vi "test-diff-drive-voltage-constraint.vi"(8 "error in (no error)":errorcluster) -> (0 "error out 4":errorcluster, 3 "Test Passed":bool)   [LabVIEW 2019]
uses:
  <vilib>/Rock Robotics/WPI/ThirdParty/JAS_Junk/TrajLib/POSE2D.ctl
  <vilib>/Rock Robotics/WPI/ThirdParty/JAS_Junk/TrajLib/TRANSLATION2D.ctl
  <vilib>/Rock Robotics/WPI/ThirdParty/JAS_Junk/TrajLib/ROTATION2D.ctl
  <vilib>/Rock Robotics/WPI/ThirdParty/JAS_Junk/TrajLib/TRAJECTORY_SPLINE_TYPE_ENUM.ctl
  <vilib>/Rock Robotics/WPI/ThirdParty/JAS_Junk/TrajLib/Translation_Create.vi
  <vilib>/Rock Robotics/WPI/ThirdParty/JAS_Junk/TrajLib/Rotation_CreateAngle.vi
  <vilib>/Rock Robotics/SystemInterfaces/NetworkCommunication/NetComm_UsageReport_report.vi
  <vilib>/Rock Robotics/WPI/ThirdParty/JAS_Junk/TrajLib/DiffDriveVoltageConstraint_New.vi
  <vilib>/Rock Robotics/WPI/ThirdParty/JAS_Junk/TrajLib/Util_LibraryGlobals.vi
  <vilib>/Rock Robotics/WPI/ThirdParty/JAS_Junk/TrajLib/Trajectory_Library.lvlib
panel:
  out "Accl Limit":dbl
  out "Abs chassis Accel":cluster{dbl[], dbl[]}[](graph)
  out "error out 3":errorcluster
  out "error out 2":errorcluster
  in  "Max Voltage-Test2":dbl=10.0 format="%#_13g"
  out "Motor VOltage Vs Time":cluster{dbl[], dbl[]}[](graph)
  in  "Max Voltage":dbl=10.0 format="%#_13g"
  out "Min Right":dbl
  out "min Left":dbl
  out "Left <":bool
  out "Left >":bool
  out "Right <":bool
  out "Right >":bool
  out "Max Right":dbl
  out "max Left":dbl
  out "Position Graph":cluster{dbl[], dbl[]}[](graph)
  out "Waypoints":T1[](array[typedef]) {"ROTATION"."SIN" format="%13.4f"; "ROTATION"."COS" format="%13.4f"; "ROTATION"."VALUE" format="%13.4f"; "TRANSLATION"."Y" format="%14.3f"; "TRANSLATION"."X" format="%14.3f"}
  out "TotalTImeSecs":dbl
  out "Error":bool
  out "error out":errorcluster
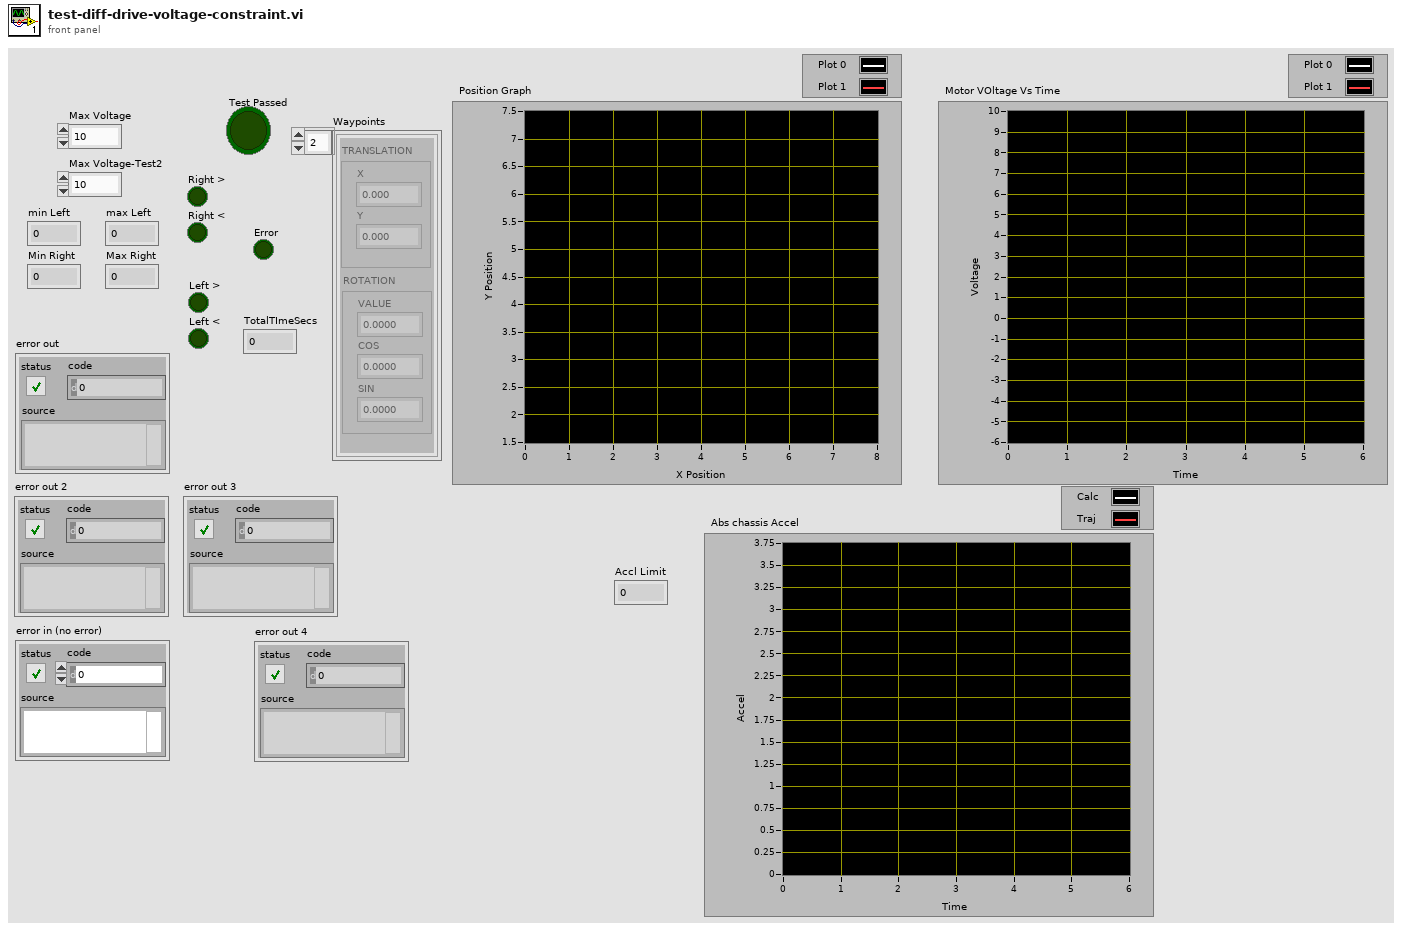
[diagram p1: front panel]
types:
  T1 = typedef "Trajectory_Library.lvlib/POSE2D.ctl" = cluster{"TRANSLATION":T2, "ROTATION":T3}
  T2 = typedef "Trajectory_Library.lvlib/TRANSLATION2D.ctl" = cluster{"X":dbl, "Y":dbl}
  T3 = typedef "Trajectory_Library.lvlib/ROTATION2D.ctl" = cluster{"VALUE":dbl, "COS":dbl, "SIN":dbl}
  T4 = typedef "Trajectory_Library.lvlib/TRAJECTORY_SPLINE_TYPE_ENUM.ctl" = enum16{"Cubic", "Cubic With Weights", "Quintic", "Quintic With Weights"}
  T5 = typedef "Trajectory_Library.lvlib/TRAJ_CONFIG.ctl" = cluster{"MaxVelocity":dbl, "Max Acceleration":dbl, "StartVelocity":dbl, "End Velocity":dbl, "Reversed":bool, "DiffDrKineConstntDefined":bool, "CentAcellConstntDefined":bool, "DiffDrVoltConstntDefined":bool, "DIFF_DRIVE_KINE_CONSTRAINT":T6, "CENTRIPETAL_ACCEL_CONSTRAINT":T8, "SwerveDrKineConstntDefined":bool, "SWERVE_DRIVE_KINE_CONSTRAINT":T9, "DIFF_DRIVE_VOLTAGE_CONSTRAINT":T12, "MECANUM_DRIVE_KINE_CONSTRAINT":T14, "MecanumDrKineConstntDefined":bool}
  T6 = typedef "Trajectory_Library.lvlib/TRAJ_CONSTRAINT_DIIF_DRIVE_KINEMATICS.ctl" = cluster{"Max Speed (M/S)":dbl, "DIFF_DRIVE_KINEMATICS":T7, "Max Accel (M/S2)":dbl}
  T7 = typedef "Trajectory_Library.lvlib/DIFF_DRIVE_KINEMATICS.ctl" = cluster{"TrackWidth_Meters":dbl}
  T8 = typedef "Trajectory_Library.lvlib/TRAJ_CONSTRAINT_CENTRIPETAL_ACCEL.ctl" = cluster{"Max Cent Accel":dbl}
  T9 = typedef "Trajectory_Library.lvlib/TRAJ_CONSTRAINT_SWERVE_DRIVE_KINEMATICS.ctl" = cluster{"Max Speed (M/S)":dbl, "SwerveKinematics":T10}
  T10 = typedef "Trajectory_Library.lvlib/SWERVE_DRIVE_KINEMATICS.ctl" = cluster{"NumModules":i32, "InverseKinematics":T11, "ForwardKinematics":T11, "Modules":T2[], "PrevCoR":T2}
  T11 = typedef "NI_Matrix.lvlib/RealMatrix.ctl" = dbl[][]
  T12 = typedef "Trajectory_Library.lvlib/TRAJ_CONSTRAINT_DIIF_DRIVE_VOLTAGE.ctl" = cluster{"Max Voltage":dbl, "DIFF_DRIVE_KINEMATICS":T7, "SIMPLE_MOTOR_FF":T13}
  T13 = typedef "Trajectory_Library.lvlib/SIMPLE_MOTOR_FF.ctl" = cluster{"Ks":dbl, "Kv":dbl, "Ka":dbl}
  T14 = typedef "Trajectory_Library.lvlib/TRAJ_CONSTRAINT_MECA_DRIVE_KINEMATICS.ctl" = cluster{"Max Speed (M/S)":dbl, "MECA_DRIVE_KINEMATICS":T15}
  T15 = typedef "Trajectory_Library.lvlib/MECA_DRIVE_KINEMATICS.ctl" = cluster{"FrontLeft":T2, "FrontRight":T2, "RearLeft":T2, "RearRight":T2, "InverseKinematics":T11, "ForwardKinematics":T11, "PrevCoR":T2}
  T16 = typedef "Trajectory_Library.lvlib/WEIGHTED_WAYPOINT.ctl" = cluster{"TRANSLATION":T2, "ROTATION":T3, "SCALAR":dbl}
  T17 = typedef "Trajectory_Library.lvlib/TRAJECTORY.ctl" = cluster{"TotalTImeSecs":dbl, "States":T18[]}
  T18 = typedef "Trajectory_Library.lvlib/TRAJ_STATE.ctl" = cluster{"TimeSeconds":dbl, "Velocity":dbl, "Acceleration":dbl, "POSE":T1, "Curvature":dbl}
  T19 = typedef "Trajectory_Library.lvlib/CHASSIS_SPEEDS.ctl" = cluster{"vX":dbl, "vY":dbl, "vOmega":dbl}
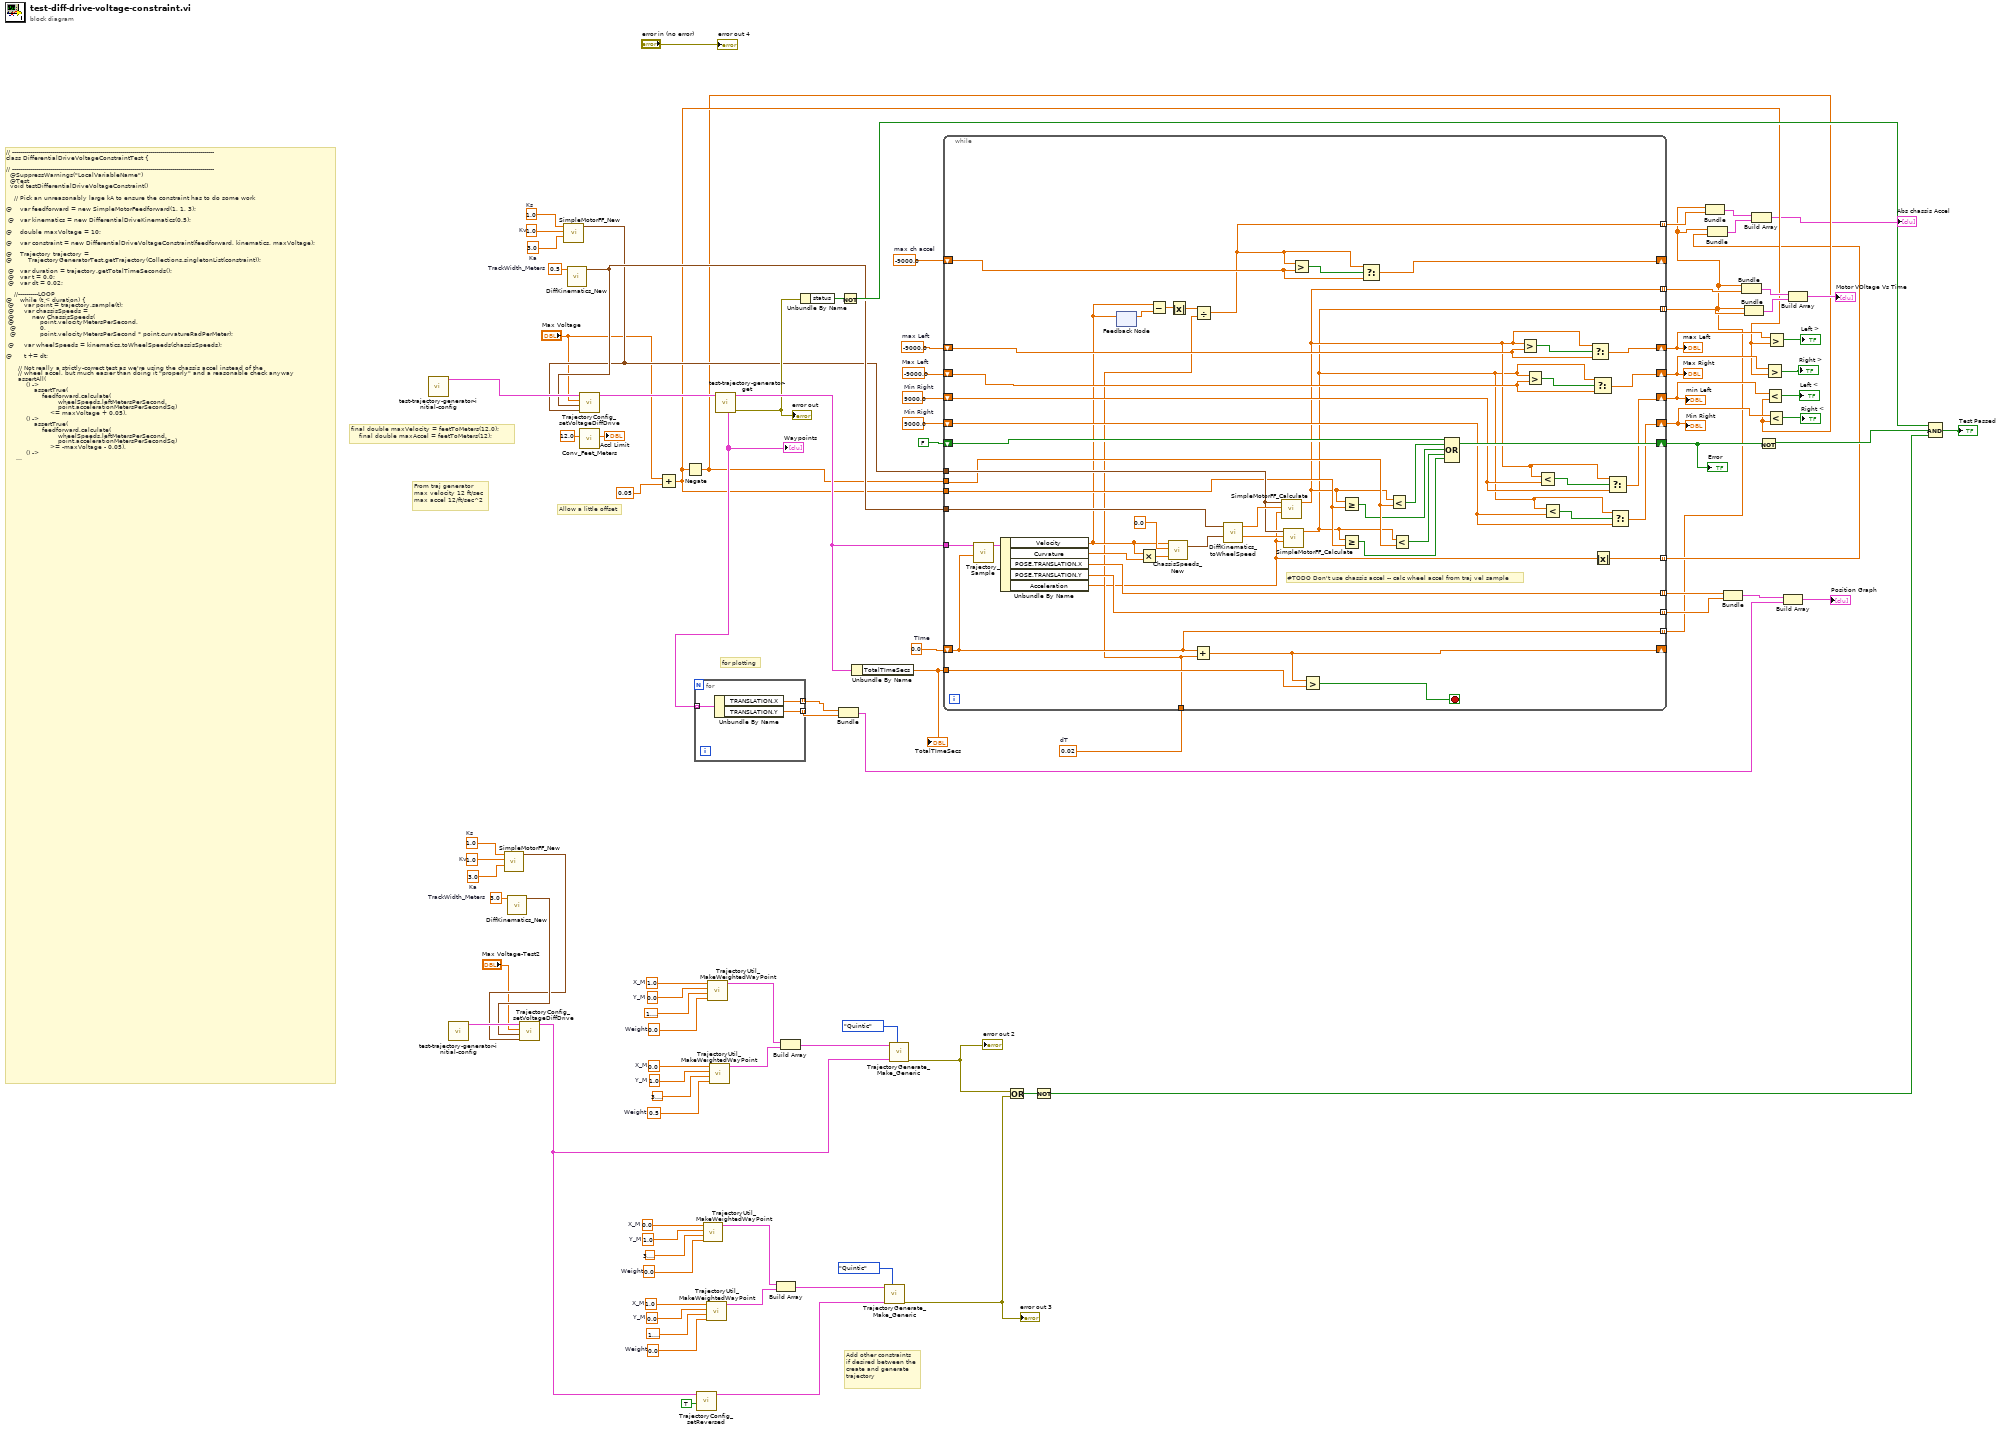
[diagram p0: block diagram]
diagram:
  w9 = -9000.0  # max ch accel
  w32 = 1.0  # X_M
  w31 = 0.0  # Y_M
  w30 = 0.0  # Weight
  w29 = 0.0  # X_M
  w28 = 1.0  # Y_M
  w27 = 0.0  # Weight
  w41 = 0.0  # X_M
  w40 = 1.0  # Y_M
  w39 = 0.5  # Weight
  w38 = 1.0  # X_M
  w37 = 0.0  # Y_M
  w36 = 0.0  # Weight
  w46 = 3.0  # TrackWidth_Meters
  w47 = 1.0  # Ks
  w48 = 1.0  # Kv
  w49 = 3.0  # Ka
  w66 = 9000.0  # Min Right
  w65 = 9000.0  # Min Right
  w72 = 0.5  # TrackWidth_Meters
  w73 = 1.0  # Ks
  w74 = 1.0  # Kv
  w75 = 3.0  # Ka
  w82 = -9000.0  # max Left
  w83 = -9000.0  # Max Left
  w95 = 0.02  # dT
  w97 = 0.0  # TIme
  # "Add other constraints\nif desired between the\ncreate and generate\ntrajectory"
  # "for plotting"
  # "final double maxVelocity = feetToMeters(12.0);\n    final double maxAccel = feetToMeters(12);"
  # "// -----------------------------------------------------------------------------------------------------\nclass DifferentialDriveVoltageConstraintTest {\n\n// -----------------------------------------------------------------------------------------------------\n  @SuppressWarnings(\"LocalVariableName\")\n  @Test\n  void testDifferentialDriveVoltageConstraint() \n\n    // Pick an unreasonably large kA to ensure the constraint has to do some work\n\n@    var feedforward = new SimpleMotorFeedforward(1, 1, 3);\n\n @   var kinematics = new DifferentialDriveKinematics(0.5);\n\n@    double maxVoltage = 10;\n\n@    var constraint = new DifferentialDriveVoltageConstraint(feedforward, kinematics, maxVoltage);\n\n@    Trajectory trajectory =\n@        TrajectoryGeneratorTest.getTrajectory(Collections.singletonList(constraint));\n\n @   var duration = trajectory.getTotalTimeSeconds();\n @   var t = 0.0;\n @   var dt = 0.02;\n\n    //----------LOOP\n@    while (t < duration) {\n @     var point = trajectory.sample(t);\n @     var chassisSpeeds =\n @         new ChassisSpeeds(\n @             point.velocityMetersPerSecond,\n  @            0,\n  @            point.velocityMetersPerSecond * point.curvatureRadPerMeter);\n\n @     var wheelSpeeds = kinematics.toWheelSpeeds(chassisSpeeds);\n\n@      t += dt;\n\n      // Not really a strictly-correct test as we're using the chassis accel instead of the\n      // wheel accel, but much easier than doing it \"properly\" and a reasonable check anyway\n      assertAll(\n          () ->\n              assertTrue(\n                  feedforward.calculate(\n                          wheelSpeeds.leftMetersPerSecond, \n                          point.accelerationMetersPerSecondSq)\n                      <= maxVoltage + 0.05),\n          () ->\n              assertTrue(\n                  feedforward.calculate(\n                          wheelSpeeds.leftMetersPerSecond, \n                          point.accelerationMetersPerSecondSq)\n                      >= -maxVoltage - 0.05),\n          () ->\n              assertTrue(\n                  feedforward.calculate(\n                          wheelSpeeds.rightMetersPerSecond, point.accelerationMetersPerSecondSq)\n                      <= maxVoltage + 0.05),\n          () ->\n              assertTrue(\n                  feedforward.calculate(\n                          wheelSpeeds.rightMetersPerSecond, point.accelerationMetersPerSecondSq)\n                      >= -maxVoltage - 0.05));\n    }  // --------END LOOP\n  }\n\n// -----------------------------------------------------------------------------------------------------\n  @Test\n  void testEndpointHighCurvature() \n\n    var feedforward = new SimpleMotorFeedforward(1, 1, 3);\n\n    // Large trackwidth - need to test with radius of curvature less than half of trackwidth\n    var kinematics = new DifferentialDriveKinematics(3);\n\n    double maxVoltage = 10;\n    var constraint = new DifferentialDriveVoltageConstraint(feedforward, kinematics, maxVoltage);\n\n    var config = new TrajectoryConfig(12, 12).addConstraint(constraint);\n\n    // Radius of curvature should be ~1 meter.\n    assertDoesNotThrow(\n        () ->\n            TrajectoryGenerator.generateTrajectory(\n                new Pose2d(1, 0, Rotation2d.fromDegrees(90)),\n                new ArrayList<Translation2d>(),\n                new Pose2d(0, 1, Rotation2d.fromDegrees(180)),\n                config));\n\n    assertDoesNotThrow(\n        () ->\n            TrajectoryGenerator.generateTrajectory(\n                new Pose2d(0, 1, Rotation2d.fromDegrees(180)),\n                new ArrayList<Translation2d>(),\n                new Pose2d(1, 0, Rotation2d.fromDegrees(90)),\n                config.setReversed(true)));\n  }\n}"
  # "Allow a little offset"
  # "From traj generator\nmax velocity 12 ft/sec\nmax accel 12/ft/sec^2"
  n1 = call "test-trajectory-generator-initial-config.vi"() -> ("traj_config"=w71:T5)  [unwired: 11 in]
  n2 = call "test-trajectory-generator-initial-config.vi"() -> ("traj_config"=w45:T5)  [unwired: 11 in]
  n3 = call <vilib>:"SimpleMotorFF_New.vi"("Ka"=w49, "Kv"=w48, "Ks"=w47) -> ("SIMPLE_MOTOR_FF"=w43:T13)  [unwired: 8 in]
  n4 = call <vilib>:"DiffKinematics_New.vi"("TrackWidth_Meters"=w46) -> ("DIFF_DRIVE_KINEMATICS"=w44:T7)  [unwired: 10 in]
  n5 = call <vilib>:"TrajectoryConfig_setVoltageDiffDrive.vi"("SIMPLE_MOTOR_FF"=w43, "DIFF_DRIVE_KINEMATICS"=w44, "Max Voltage"="Max Voltage-Test2", "inTRAJECTORY_CONFIG"=w45) -> ("outTRAJECTORY_CONFIG"=w13:T5)  [unwired: 7 in]
  n6 = call <vilib>:"SimpleMotorFF_New.vi"("Ka"=w75, "Kv"=w74, "Ks"=w73) -> ("SIMPLE_MOTOR_FF"=w68:T13)  [unwired: 8 in]
  n7 = call <vilib>:"DiffKinematics_New.vi"("TrackWidth_Meters"=w72) -> ("DIFF_DRIVE_KINEMATICS"=w69:T7)  [unwired: 10 in]
  n8 = call <vilib>:"TrajectoryConfig_setVoltageDiffDrive.vi"("SIMPLE_MOTOR_FF"=w68, "DIFF_DRIVE_KINEMATICS"=w69, "Max Voltage"="Max Voltage", "inTRAJECTORY_CONFIG"=w71) -> ("outTRAJECTORY_CONFIG"=w70:T5)  [unwired: 7 in]
  n9 = call <vilib>:"Conv_Feet_Meters.vi"("Feet"=12.0) -> ("Meters"=→"Accl Limit":dbl)  [unwired: 10 in]
  n10 = Add(x="Max Voltage", y=0.05) -> (x+y=w53:dbl)
  n11 = Negate(x=w53) -> (-x=w50:dbl)
  n12 = call <vilib>:"TrajectoryConfig_setReversed.vi"("Reversed"=TRUE, "inTRAJECTORY_CONFIG"=w13) -> ("outTRAJECTORY_CONFIG"=w11:T5)  [unwired: 9 in]
  n13 = call <vilib>:"TrajectoryUtil_MakeWeightedWayPoint.vi"("Weight"=w27, "Travel Angle Radians"=3.141592653589793, "Y_M"=w28, "X_M"=w29) -> ("WEIGHTED_WAYPOINT"=w24:T16)  [unwired: 7 in]
  n14 = call <vilib>:"TrajectoryUtil_MakeWeightedWayPoint.vi"("Weight"=w30, "Travel Angle Radians"=1.5707963267948966, "Y_M"=w31, "X_M"=w32) -> ("WEIGHTED_WAYPOINT"=w20:T16)  [unwired: 7 in]
  n15 = call <vilib>:"TrajectoryUtil_MakeWeightedWayPoint.vi"("Weight"=w36, "Travel Angle Radians"=1.5707963267948966, "Y_M"=w37, "X_M"=w38) -> ("WEIGHTED_WAYPOINT"=w33:T16)  [unwired: 7 in]
  n16 = call <vilib>:"TrajectoryUtil_MakeWeightedWayPoint.vi"("Weight"=w39, "Travel Angle Radians"=3.141592653589793, "Y_M"=w40, "X_M"=w41) -> ("WEIGHTED_WAYPOINT"=w23:T16)  [unwired: 7 in]
  n17 = call "test-trajectory-generator-get.vi"("traj_config"=w70) -> ("error out"=w78:errorcluster, "TRAJECTORY"=w94:T17, "Waypoints"=w91:T1[])  [unwired: 8 in]
  "error out" <- w78
  "Waypoints" <- w91
  n18 = for {
    tunnel: w91 -> [w100] mode=indexing
    tunnel: [w99] -> w90 mode=indexing
    tunnel: [w98] -> w89 mode=indexing
    n19 = Unbundle By Name(w100) -> ("TRANSLATION.X"=w99:dbl, "TRANSLATION.Y"=w98:dbl)
  }
  n20 = Build Array(w24, w20) -> (w25:T16[])
  n21 = Build Array(w33, w23) -> (w34:T16[])
  n22 = Unbundle By Name(w78) -> ("status"=w77:bool)
  n23 = Bundle(w90, w89) -> (w85:cluster{dbl[], dbl[]})  [unwired: 1 in]
  n24 = Not(x=w77) -> (.not. x?=w76:bool)
  n25 = Unbundle By Name(w94) -> ("TotalTImeSecs"=w96:dbl)
  "TotalTImeSecs" <- w96
  n26 = call <vilib>:"TrajectoryGenerate_Make_Generic.vi"("Spline Type"=TRAJECTORY_SPLINE_TYPE_ENUM."Quintic", "traj_config"=w11, "WeightedWayPoints"=w25) -> ("error out"=w15:errorcluster)  [unwired: 7 in, 1 out]
  "error out 3" <- w15
  n27 = call <vilib>:"TrajectoryGenerate_Make_Generic.vi"("Spline Type"=TRAJECTORY_SPLINE_TYPE_ENUM."Quintic", "traj_config"=w13, "WeightedWayPoints"=w34) -> ("error out"=w16:errorcluster)  [unwired: 7 in, 1 out]
  "error out 2" <- w16
  n28 = while {
    tunnel: w96 -> [w148]
    shift-right: [w149] -> _
    shift-left: w97 -> [w112]
    tunnel: w95 -> [w107]
    tunnel: w94 -> [w146]
    shift-right: [w139] -> w79
    shift-left: FALSE -> [w140]
    tunnel: w50 -> [w125]
    tunnel: [w138] -> w88 mode=indexing
    tunnel: [w137] -> w87 mode=indexing
    shift-right: [w135] -> w57
    shift-left: w82 -> [w134]
    shift-right: [w136] -> w56
    shift-left: w83 -> [w133]
    tunnel: w69 -> [w130]
    tunnel: w68 -> [w127]
    tunnel: w53 -> [w124]
    shift-right: [w118] -> w55
    shift-left: w66 -> [w116]
    shift-right: [w117] -> w54
    shift-left: w65 -> [w115]
    tunnel: [w114] -> w64 mode=indexing
    tunnel: [w113] -> w63 mode=indexing
    tunnel: [w112] -> w4 mode=indexing
    shift-right: [w104] -> _
    shift-left: w9 -> [w105]
    tunnel: [w101] -> w6 mode=indexing
    tunnel: [w103] -> w5 mode=indexing
    stop <- w147 stop-if-true
    # "#TODO Don't use chassis accel -- calc wheel accel from traj vel sample"
    n29 = call <vilib>:"Trajectory_Sample.vi"("Time"=w112, "InputTRAJECTORY"=w146) -> ("OutputTRAJ_STATE"=w145:T18)  [unwired: 9 in]
    n30 = Unbundle By Name(w145) -> ("Velocity"=w110:dbl, "Curvature"=w142:dbl, "POSE.TRANSLATION.X"=w138:dbl, "POSE.TRANSLATION.Y"=w137:dbl, "Acceleration"=w102:dbl)
    n31 = feedback-in #1(w110) -> ()
    n32 = feedback #1() -> (w111:dbl)  [unwired: 1 in]
    n33 = Multiply(x=w110, y=w142) -> (x*y=w143:dbl)
    n34 = Subtract(x=w110, y=w111) -> (x-y=w109:dbl)
    n35 = call <vilib>:"ChassisSpeeds_New.vi"("vAngular"=w143, "vY"=0.0, "vX"=w110) -> ("CHASSIS"=w141:T19)  [unwired: 8 in]
    n36 = Absolute Value(x=w109) -> (abs(x)=w108:dbl)
    n37 = Add(x=w112, y=w107) -> (x+y=w149:dbl)
    n38 = Divide(x=w108, y=w107) -> (x/y=w103:dbl)
    n39 = call <vilib>:"DiffKinematics_toWheelSpeed.vi"("CHASSIS Speed"=w141, "DIFF_DRIVE_KINEMATICS"=w130) -> ("RightVelocity"=w129:dbl, "LeftVelocity"=w128:dbl)  [unwired: 8 in]
    n40 = call <vilib>:"SimpleMotorFF_Calculate.vi"("Accel"=w102, "Vel"=w128, "SIMPLE_MOTOR_FF"=w127) -> ("FeedForward"=w114:dbl)  [unwired: 8 in]
    n41 = call <vilib>:"SimpleMotorFF_Calculate.vi"("Accel"=w102, "Vel"=w129, "SIMPLE_MOTOR_FF"=w127) -> ("FeedForward"=w113:dbl)  [unwired: 8 in]
    n42 = Greater?(x=w103, y=w105) -> (0:w106:bool)
    n43 = Greater?(x=w149, y=w148) -> (0:w147:bool)
    n44 = Greater Or Equal?(x=w114, y=w124) -> (x >= y?=w122:bool)
    n45 = Greater Or Equal?(x=w113, y=w124) -> (x >= y?=w126:bool)
    n46 = Select(t=w103, s=w106, f=w105) -> (s? t:f=w104:dbl)
    n47 = Less?(x=w114, y=w125) -> (x < y?=w121:bool)
    n48 = Less?(x=w113, y=w125) -> (x < y?=w123:bool)
    n49 = Compound Arithmetic op=OR(w140, w121, w122, w123, w126) -> (w139:bool)
    n50 = Greater?(x=w114, y=w134) -> (0:w132:bool)
    n51 = Greater?(x=w113, y=w133) -> (0:w131:bool)
    n52 = Less?(x=w114, y=w116) -> (x < y?=w120:bool)
    n53 = Less?(x=w113, y=w115) -> (x < y?=w119:bool)
    n54 = Select(t=w114, s=w132, f=w134) -> (s? t:f=w135:dbl)
    n55 = Select(t=w113, s=w131, f=w133) -> (s? t:f=w136:dbl)
    n56 = Absolute Value(x=w102) -> (abs(x)=w101:dbl)
    n57 = Select(t=w114, s=w120, f=w116) -> (s? t:f=w118:dbl)
    n58 = Select(t=w113, s=w119, f=w115) -> (s? t:f=w117:dbl)
  }
  "Error" <- w79
  "max Left" <- w57
  "Max Right" <- w56
  "min Left" <- w55
  "Min Right" <- w54
  n59 = Or(x=w16, y=w15) -> (x .or. y?=w17:bool)
  n60 = Not(x=w17) -> (.not. x?=w14:bool)
  n61 = Bundle(w4, w5) -> (w8:cluster{dbl[], dbl[]})  [unwired: 1 in]
  n62 = Bundle(w4, w6) -> (w7:cluster{dbl[], dbl[]})  [unwired: 1 in]
  n63 = Bundle(w88, w87) -> (w86:cluster{dbl[], dbl[]})  [unwired: 1 in]
  n64 = Bundle(w4, w64) -> (w61:cluster{dbl[], dbl[]})  [unwired: 1 in]
  n65 = Bundle(w4, w63) -> (w60:cluster{dbl[], dbl[]})  [unwired: 1 in]
  n66 = Build Array(w8, w7) -> (→"Abs chassis Accel":cluster{dbl[], dbl[]}[])
  n67 = Not(x=w79) -> (.not. x?=w80:bool)
  n68 = Greater?(x=w56, y=w53) -> (0:→"Right >":bool)
  n69 = Less?(x=w55, y=w50) -> (x < y?=→"Left <":bool)
  n70 = Less?(x=w54, y=w50) -> (x < y?=→"Right <":bool)
  n71 = Greater?(x=w57, y=w53) -> (0:→"Left >":bool)
  n72 = Build Array(w86, w85) -> (→"Position Graph":cluster{dbl[], dbl[]}[])
  n73 = Build Array(w61, w60) -> (→"Motor VOltage Vs Time":cluster{dbl[], dbl[]}[])
  n74 = Compound Arithmetic op=AND(w76, w80, w14) -> (→"Test Passed":bool)
  "error out 4" <- "error in (no error)"
